vi "add item and setting.vi"(8 "error in (no error)":errorcluster, 9 "Tag":string, 10 "items":T3(array[cluster]), 11 "Application Data in":T1) -> (0 "error out":errorcluster, 2 "new item tag":string, 3 "Application Data out":T1)   [LabVIEW 2017]
uses:
  Application Data.ctl
  DSF Configuration API/1.0.0/Public/Controls/DSF Config Data RefNum.ctl
  Window State.ctl
  DSF Configuration API/1.0.0/DSF Configuration API.lvlib
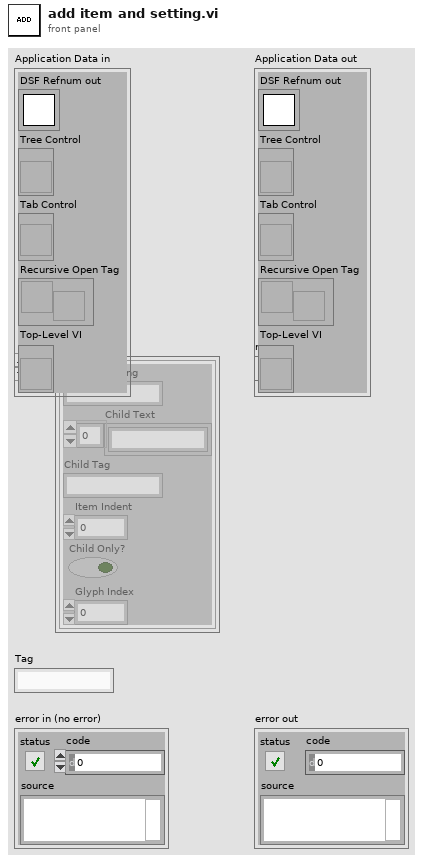
[diagram p1: front panel]
types:
  T1 = typedef "Application Data.ctl" = cluster{"DSF Refnum out":T2, "Tree Control":refnum<vi>, "Tab Control":refnum<vi>, "Recursive Open Tag":refnum<user-event>, "Top-Level VI":refnum<vi>}
  T2 = typedef "DSF Configuration API.lvlib/DSF Config Data RefNum.ctl" = refnum<k1>
  T3 = cluster{"Left Cell String":string, "Child Text":string[], "Child Tag":string, "Item Indent":i32, "Child Only?":bool, "Glyph Index":i32}[]
  T4 = cluster{"Left Cell String":string, "Child Text":string[], "Child Tag":string, "Item Indent":i32, "Child Only?":bool, "Glyph Index":i32}
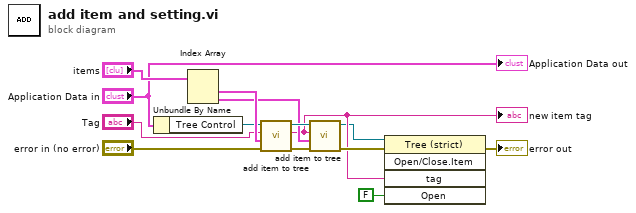
[diagram p0: block diagram]
diagram:
  n1 = Unbundle By Name("Application Data in") -> ("Tree Control"=w1:refnum<vi>)
  n2 = Index Array(array="items") -> (element #1=w13:T4, element #2=w10:T4)  [unwired: 2 in]
  n3 = call "add item to tree.vi"("error in (no error)"="error in (no error)", "Item"=w13, "display name"="Tag", "TreeControl in"=w1) -> ("error out"=w11:errorcluster, "new item tag"=w8:string, "TreeControl out"=w12:refnum<vi>)  [unwired: 5 in]
  "new item tag" <- w8
  n4 = call "add item to tree.vi"("error in (no error)"=w11, "Item"=w10, "display name"=w8, "TreeControl in"=w12) -> ("error out"=w9:errorcluster, "TreeControl out"=w7:refnum<vi>)  [unwired: 5 in, 1 out]
  n5 = invoke class="Tree (strict)" method="Open/Close.Item"(reference=w7, error in=w9, "tag"=w8, "Open"=FALSE ("Open?")) -> (error out=→"error out":errorcluster)  [unwired: 1 in, 4 out]
  "Application Data out" <- "Application Data in"
